vi "ERP42 PC_Program수정_2.vi"() -> ()   [LabVIEW 2018]
uses:
  <vilib>/Instr/_visa.llb/VISA Configure Serial Port (Instr).vi
  Global brake.vi
  Global speed.vi
panel:
  in  "Brake_CMD":u8(slide)=1 min=1 max=200 step=1 scale=1.0..200.0
  out "브레이크":u8
  out "조향":i16
  out "속도":u8
  out "Alive":u8
  in  "GEAR_CMD":u8 max=2
  out "ALIVE":u8
  out "Encoder":u8
  in  "E-STOP_CMD":bool
  in  "M/A_CMD":bool
  in  "pc 연결(com3)":refnum<visa-resource-name> caption="UPPER"
  out "BRAKE":i16
  out "STEER":i16
  out "SPEED":u8
  out "GEAR":u8
  out "E-STOP":u8
  out "M/A":u8
  out "Data Read":string
  in  "stop":bool
  # "brake : 100 (full)"
  # "ERP42 PC Program"
  # "ERP42 Data CMD"
  # "ERP42 Data Receive"
  # "좌"
  # "우"
  # "좌"
  # "우"
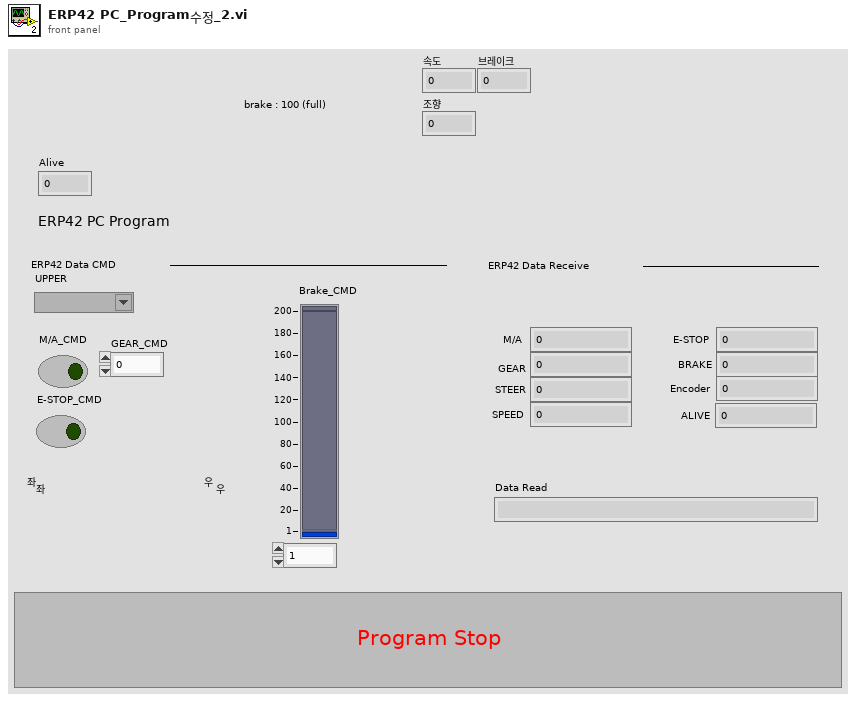
[diagram p1: front panel]
types:
  T1 = typedef "컨트롤 1.ctl" = cluster{"M/A":u8, "Speed":u16, "Steer":i16, "Brake":i16, "E-STOP":u8, "GEAR":u8, "ENCODER":u8, "ALIVE":u8}
  T2 = typedef "컨트롤 6.ctl" = cluster{"GEAR":u8, "Speed":u16, "Steer":i16, "Brake":i16, "M/A":u8, "E-STOP":u8, "ALIVE":u8}
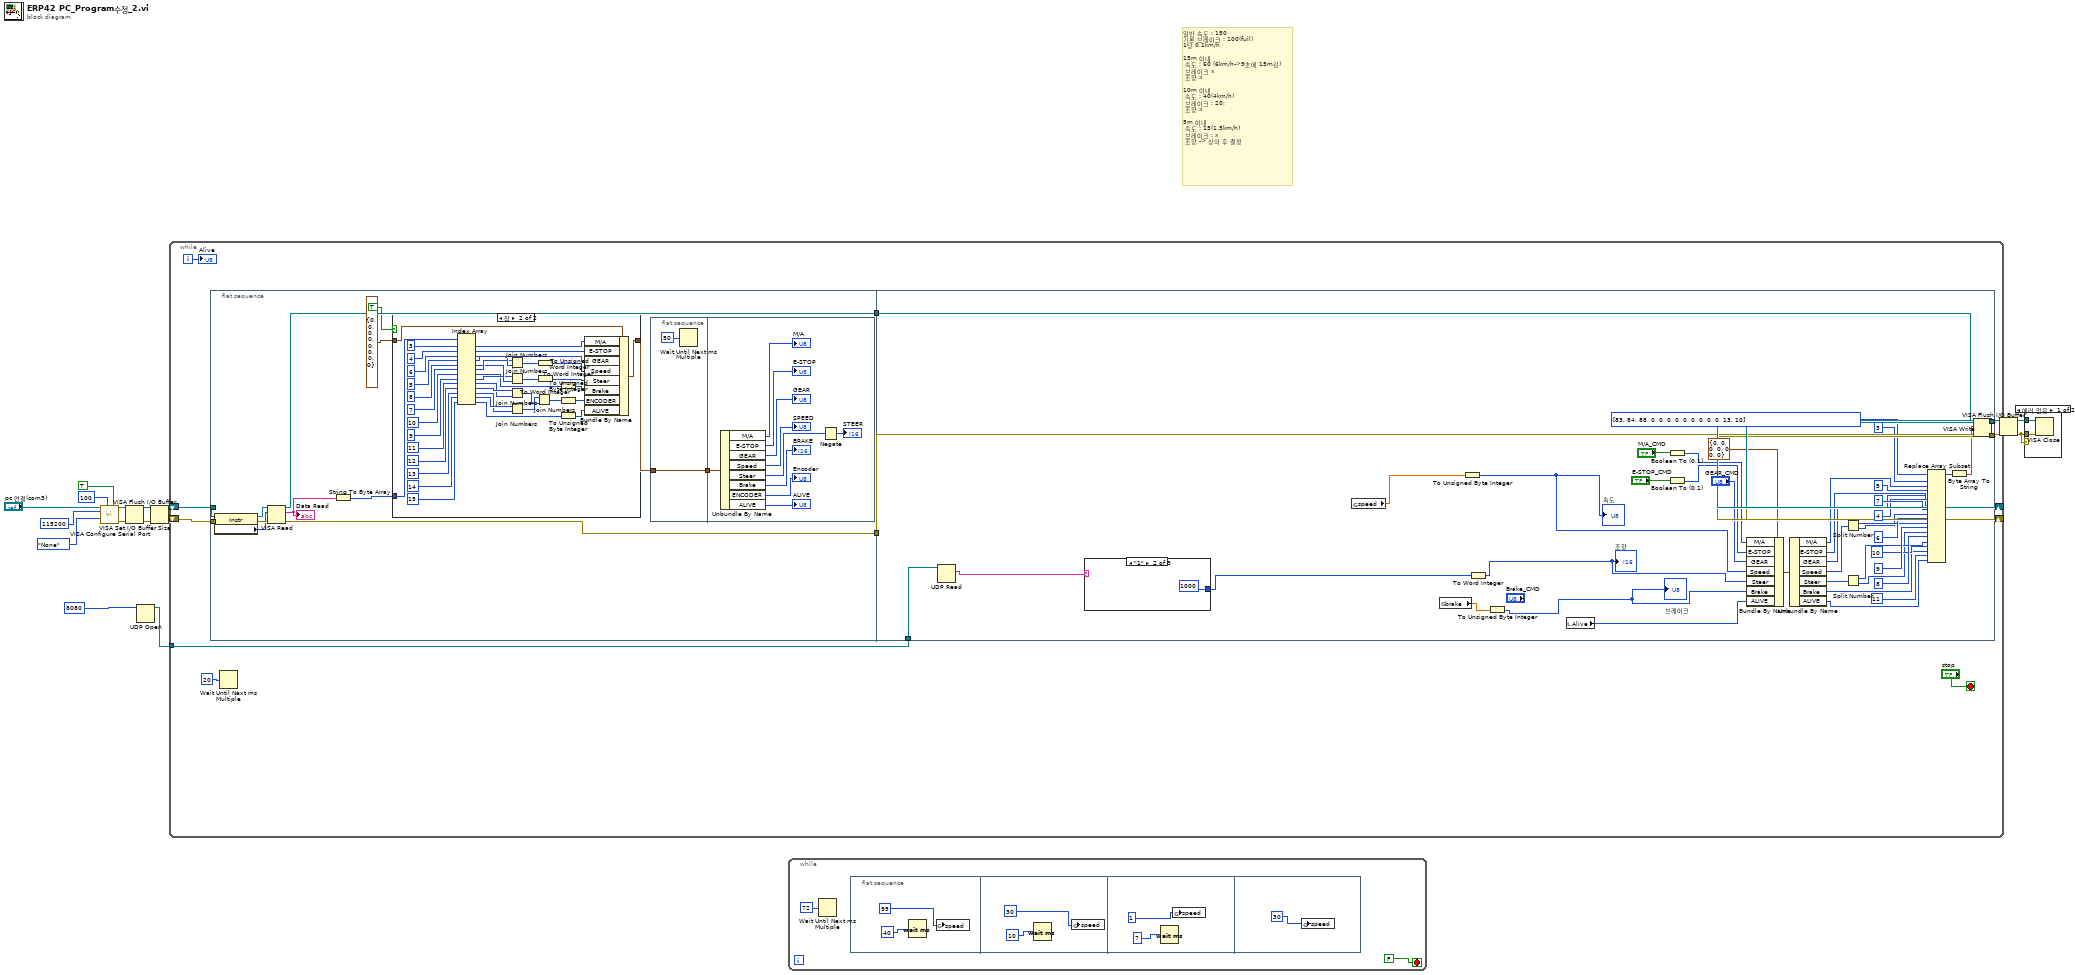
[diagram p0: block diagram]
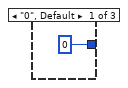
[diagram p4: hidden frame]
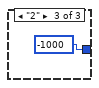
[diagram p5: hidden frame]
diagram:
  # "일반 속도 : 150\n기본 브레이크 : 100(full) \n1당 0.1km/h\n\n15m 이내 \n 속도 : 60 (6km/h->9초에 15m감)\n 브레이크 x\n 조향 x\n\n10m 이내\n 속도 : 40(4km/h)\n 브레이크 : 20;\n 조향 x\n\n5m 이내\n 속도 : 15(1.5km/h)\n 브레이크 : x\n 조향 -> 상의 후 결정"
  n1 = call-poly "VISA Configure Serial Port"("VISA resource name"="pc 연결(com3)", "timeout (10sec)"=u32 100, "Enable Termination\nChar (T)"=TRUE ("Enable Termination\nChar (T)"), "baud rate (9600)"=u32 115200, "parity (0:none)"=enum16{"None", "Odd", "Even", "Mark", "Space"}."None") -> ("VISA resource name out"=w15:refnum<visa-resource-name>, "error out"=w14:errorcluster)  [unwired: 9 in]
  n2 = VISA Set I/O Buffer Size(VISA resource name=w15, error in (no error)=w14) -> (VISA resource name out=w13:refnum<visa-resource-name>, error out=w16:errorcluster)  [unwired: 2 in]
  n3 = UDP Open(11:u16 8080 ("port")) -> (port=w1:refnum<k16>)  [unwired: 4 in, 2 out]
  n4 = VISA Flush I/O Buffer(VISA resource name=w13, error in (no error)=w16) -> (VISA resource name out=w10:refnum<visa-resource-name>, error out=w7:errorcluster)  [unwired: 1 in]
  n5 = while {
    shift-right: [w22] -> w4
    shift-left: w10 -> [w27]
    shift-right: [w21] -> w3
    shift-left: w7 -> [w26]
    tunnel: w1 -> [w18]
    i -> [w23]
    stop <- "stop" stop-if-true
    n6 = flat-sequence {
      tunnel: [w36] -> w20
      tunnel: w27 -> [w40]
      tunnel: w26 -> [w39]
      tunnel: [w30] -> w19
      tunnel: w20 -> [w135]
      tunnel: [w134] -> w22
      tunnel: w19 -> [w108]
      tunnel: [w107] -> w21
      tunnel: w18 -> [w96]
      frame #0 {
        n7 = property class="Instr"(reference=w40, error in=w39) -> (reference out=w38:refnum<visa-resource-name>, error out=w37:errorcluster, "Serial Settings:Number of Bytes at Serial Port"=w31:u32)
        n8 = VISA Read(VISA resource name=w38, byte count=w31, error in (no error)=w37) -> (VISA resource name out=w30:refnum<visa-resource-name>, read buffer=w32:string, error out=w36:errorcluster)  [unwired: 1 out]
        "Data Read" <- w32
        n9 = String To Byte Array(string=w32) -> (unsigned byte array=w33:u8[])
        n10 = case shown="참" TRUE {
          tunnel: w33 -> [_ w92]
          tunnel: [w53 w81] -> w35
          tunnel: T1 {"M/A"=0, "Speed"=0, "Steer"=0, "Brake"=0, "E-STOP"=0, "GEAR"=0, "ENCODER"=0, "ALIVE"=0} ("Protocol_Read") -> [w53 w80]
          frame False {
            # "선 연결함 -> 원래 안되있었음"
          }
          frame True {
            n11 = Index Array(array=w92, index #1=3, index #2=4, index #3=6, index #4=5, index #5=8, index #6=7, index #7=10, index #8=9, index #9=11 ("인덱스"), index #10=12 ("인덱스"), index #11=13 ("인덱스"), index #12=14 ("인덱스"), index #13=15 ("인덱스")) -> (element #1=w83:u8, element #2=w82:u8, element #3=w78:u8, element #4=w79:u8, element #5=w76:u8, element #6=w77:u8, element #7=w59:u8, element #8=w75:u8, element #9=w68:u8, element #10=w69:u8, element #11=w66:u8, element #12=w67:u8, element #13=w63:u8)
            n12 = Join Numbers(hi=w77, lo=w78) -> ((hi.lo)=w54:u16)
            n13 = Join Numbers(hi=w75, lo=w76) -> ((hi.lo)=w56:u16)
            n14 = Join Numbers(hi=w69, lo=w68) -> ((hi.lo)=w64:u16)
            n15 = Join Numbers(hi=w67, lo=w66) -> ((hi.lo)=w65:u16)
            n16 = Join Numbers(hi=w65, lo=w64) -> ((hi.lo)=w61:u32)
            n17 = To Unsigned Word Integer(number=w54) -> (unsigned 16bit integer=w55:u16)
            n18 = To Word Integer(number=w56) -> (16bit integer=w57:i16)
            n19 = To Word Integer(number=w59) -> (16bit integer=w58:i16)
            n20 = To Unsigned Byte Integer(number=w61) -> (unsigned 8bit integer=w60:u8)
            n21 = To Unsigned Byte Integer(number=w63) -> (unsigned 8bit integer=w62:u8)
            n22 = Bundle By Name(cluster=w80, "M/A"=w83, "E-STOP"=w82, "GEAR"=w79, "Speed"=w55, "Steer"=w57, "Brake"=w58, "ENCODER"=w60, "ALIVE"=w62) -> (w81:T1)
          }
        }
        n23 = flat-sequence {
          tunnel: w35 -> [w42]
          tunnel: [w42] -> w28
          tunnel: w28 -> [w52]
          frame #0 {
            n24 = Wait Until Next ms Multiple(millisecond multiple=i16 50) -> ()  [unwired: 1 out]
          }
          frame #1 {
            n25 = Unbundle By Name(w52) -> ("M/A"=→"M/A":u8, "E-STOP"=→"E-STOP":u8, "GEAR"=→"GEAR":u8, "Speed"=→"SPEED":u16, "Steer"=w43:i16, "Brake"=→"BRAKE":i16, "ENCODER"=→"Encoder":u8, "ALIVE"=→"ALIVE":u8)
            n26 = Negate(x=w43) -> (-x=→"STEER":i16)
          }
        }
      }
      frame #1 {
        n27 = UDP Read(connection ID=w96) -> (data out=w95:string)  [unwired: 3 in, 4 out]
        n28 = case shown="\"1\"" w95 {
          tunnel: [0 1000 -1000] -> w94
          frame "0", Default {
          }
          frame "1" {
          }
          frame "2" {
          }
        }
        n29 = global read "Global speed.vi" "speed"() -> (w93:dbl)
        n30 = global read "Global brake.vi" "brake"() -> (w98:dbl)
        n31 = To Unsigned Byte Integer(number=w93) -> (unsigned 8bit integer=w100:u8)
        "속도" <- w100
        n32 = To Word Integer(number=w94) -> (16bit integer=w99:i16)
        "조향" <- w99
        n33 = To Unsigned Byte Integer(number=w98) -> (unsigned 8bit integer=w97:u8)
        "브레이크" <- w97
        n34 = local read "Alive"() -> (w104:u8)
        n35 = Boolean To (0,1)(Boolean="M/A_CMD") -> (0, 1=w123:i16)
        n36 = Boolean To (0,1)(Boolean="E-STOP_CMD") -> (0, 1=w118:i16)
        n37 = Bundle By Name(cluster=T2 {"GEAR"=0, "Speed"=0, "Steer"=0, "Brake"=0, "M/A"=0, "E-STOP"=0, "ALIVE"=0} ("Protocol_Write"), "M/A"=w123, "E-STOP"=w118, "GEAR"="GEAR_CMD", "Speed"=w100, "Steer"=w99, "Brake"=w97, "ALIVE"=w104) -> (w121:T2)
        n38 = Unbundle By Name(w121) -> ("M/A"=w117:u8, "E-STOP"=w116:u8, "GEAR"=w115:u8, "Speed"=w114:u16, "Steer"=w113:i16, "Brake"=w112:i16, "ALIVE"=w109:u8)
        n39 = Split Number(x=w114) -> (hi(x)=w102:u8, lo(x)=w101:u8)
        n40 = Split Number(x=w113) -> (hi(x)=w106:u8, lo(x)=w105:u8)
        n41 = Replace Array Subset(array=u8[] [83, 84, 88, 0, 0, 0, 0, 0, 0, 0, 0, 0, 13, 10] ("unsigned byte array"), new element #1=w117, index #1=3, new element #2=w115, index #2=5, new element #3=w116, index #3=4, new element #4=w101, index #4=7, new element #5=w102, index #5=6, new element #6=w105, index #6=9, new element #7=w106, index #7=8, new element #8=w112, index #8=10, new element #9=w109, index #9=11 ("인덱스")) -> (w103:u8[])
        n42 = Byte Array To String(unsigned byte array=w103) -> (string=w125:string)
        n43 = VISA Write(VISA resource name=w108, write buffer=w125, error in (no error)=w135) -> (VISA resource name out=w134:refnum<visa-resource-name>, error out=w107:errorcluster)  [unwired: 1 out]
      }
    }
    n44 = Wait Until Next ms Multiple(millisecond multiple=i16 20) -> ()  [unwired: 1 out]
    "Alive" <- w23
  }
  n45 = while {
    stop <- FALSE ("Enable Termination\nChar (T)") stop-if-true
    n46 = Wait Until Next ms Multiple(millisecond multiple=i16 72) -> ()  [unwired: 1 out]
    n47 = flat-sequence {
      frame #0 {
        n48 = Wait (ms)(milliseconds to wait=40) -> ()  [unwired: 1 out]
        n49 = global write "Global speed.vi" "speed"(95) -> ()
      }
      frame #1 {
        n50 = Wait (ms)(milliseconds to wait=10) -> ()  [unwired: 1 out]
        n51 = global write "Global speed.vi" "speed"(30) -> ()
      }
      frame #2 {
        n52 = Wait (ms)(milliseconds to wait=7) -> ()  [unwired: 1 out]
        n53 = global write "Global speed.vi" "speed"(1) -> ()
      }
      frame #3 {
        n54 = global write "Global speed.vi" "speed"(30 ("speed")) -> ()
      }
    }
  }
  n55 = VISA Flush I/O Buffer(VISA resource name=w4, error in (no error)=w3) -> (VISA resource name out=w8:refnum<visa-resource-name>, error out=w9:errorcluster)  [unwired: 1 in]
  n56 = case shown="에러 없음" w9 {
    tunnel: w9 -> [w149 _]
    tunnel: w8 -> [w148 _]
    frame No Error {
      n57 = VISA Close(VISA resource name=w148, error in (no error)=w149) -> ()  [unwired: 1 out]
    }
    frame Error {
    }
  }
